vi "_Replace Configuration Table By ID(Element).vi"(6 "Comment Express Pattern(^#)":string="^#", 8 "Error in":errorcluster caption="Error in (no error)", 9 "ID Col":i32, 10 "New Line":string[](array[string]), 11 "Table in":string[][](array[string])) -> (0 "Error out":errorcluster, 3 "Table out":string[][](array[string]))   [LabVIEW 2017]
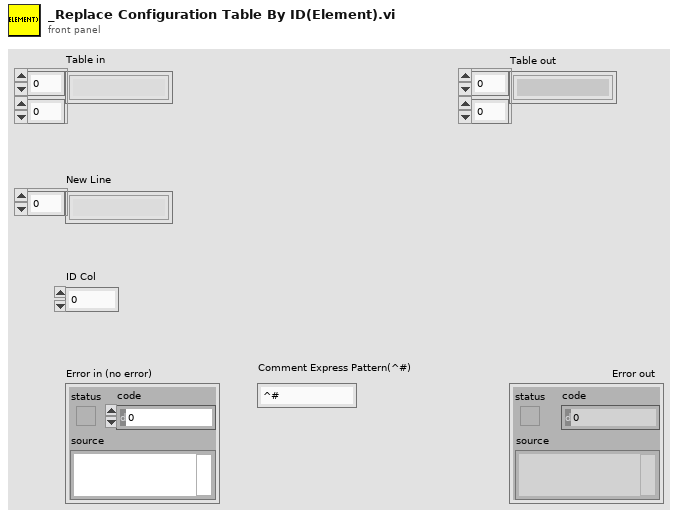
[diagram p1: front panel]
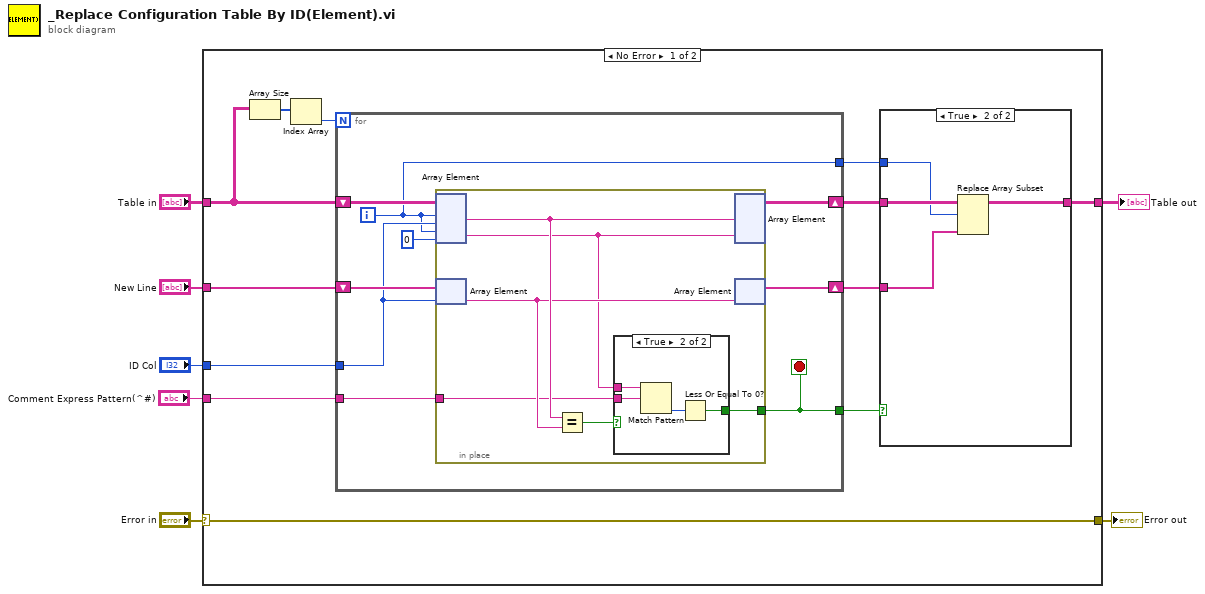
[diagram p0: block diagram]
diagram:
  n1 = case shown="No Error" "Error in" {
    selector: "Error in" -> [w8 w45]
    tunnel: "New Line" -> [w19 _]
    tunnel: "ID Col" -> [w18 _]
    tunnel: "Comment Express Pattern(^#)" -> [w16 _]
    tunnel: [w15 w44] -> w4
    tunnel: "Table in" -> [w11 w44]
    tunnel: [w8 w45] -> w1
    frame No Error {
      n2 = Array Size(array=w11) -> (size(s)=w10:i32[])
      n3 = Index Array(array=w10) -> (element=w9:i32)  [unwired: 1 in]
      n4 = for {
        N: w9 -> [_]
        tunnel: w18 -> [w30]
        shift-right: [w31] -> w17
        shift-left: w11 -> [w32]
        tunnel: w16 -> [w28]
        shift-right: [w27] -> w14
        shift-left: w19 -> [w33]
        tunnel: [w26] -> w12
        tunnel: [w25] -> w13
        i -> [w26]
        stop <- w25 stop-if-true
        n5 = in-place {
          in-place-border: w28 -> [w36]
          in-place-border: [w34] -> w25
          n6 = in-place-array #1(w32, w26, w30, w26, 0) -> (w39:string, w37:string)
          n7 = in-place-array #2(w33, w30) -> (w38:string)
          n8 = Equal?(x=w39, y=w38) -> (x = y?=w35:bool)
          n9 = case shown="True" w35 {
            tunnel: w37 -> [_ w43]
            tunnel: w36 -> [_ w42]
            tunnel: [_ w40] -> w34
            frame False {
            }
            frame True {
              n10 = Match Pattern(string=w43, regular expression=w42) -> (offset past match=w41:i32)  [unwired: 1 in, 3 out]
              n11 = Less Or Equal To 0?(x=w41) -> (x <= 0?=w40:bool)
            }
          }
          n12 = in-place-array #1(w39, w37) -> (w31:string[][])  [unwired: 4 out]
          n13 = in-place-array #2(w38) -> (w27:string[])  [unwired: 1 out]
        }
      }
      n14 = case shown="True" w13 {
        tunnel: w17 -> [w20 w24]
        tunnel: [w20 w23] -> w15
        tunnel: w14 -> [_ w22]
        tunnel: w12 -> [_ w21]
        frame False {
        }
        frame True {
          n15 = Replace Array Subset(array=w24, new element=w22, index (row)=w21) -> (w23:string[][])  [unwired: 1 in]
        }
      }
    }
    frame Error {
    }
  }
  "Table out" <- w4
  "Error out" <- w1
